vi "Is Private Data Empty.vi"(8 "error in":errorcluster, 10 "Ref.Private Data Cluster":refnum<vi>) -> (0 "error out":errorcluster, 2 "Private Data Empty?":bool)   [LabVIEW 2021, in "_Rescript Msg.lvlib" / "_Rescript Msg.lvclass"]
uses:
  _Rescript Msg.lvclass
  _Rescript Msg.lvclass/_Rescript Msg.ctl
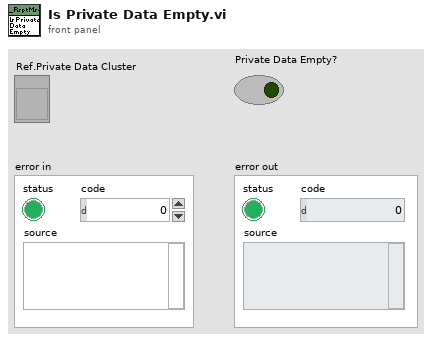
[diagram p1: front panel]
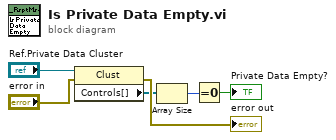
[diagram p0: block diagram]
diagram:
  n1 = property class="Clust"(reference="Ref.Private Data Cluster", error in="error in") -> (error out=→"error out":errorcluster, "Controls[]"=w3:refnum<vi>[])  [unwired: 1 out]
  n2 = Array Size(array=w3) -> (size(s)=w6:i32)
  n3 = Equal To 0?(x=w6) -> (x = 0?=→"Private Data Empty?":bool)
